vi "example_02_two_button.vi"() -> ()   [LabVIEW 2015, in "lv-dialog.lvlib" / "v1.lvlib"]
uses:
  v1.lvlib
  public/_controls/dialog_selection.ctl
  public/class/v1.lvclass
panel:
  in  "boolean_text_2":string="OK"
  in  "boolean_text_1":string="OK"
  in  "dialog_text":string="Press a button"
  out "error out":errorcluster
  out "dialog_selection":T1
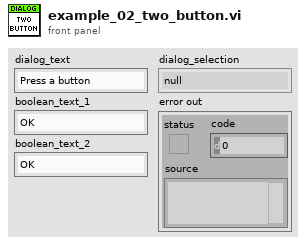
[diagram p1: front panel]
types:
  T1 = typedef "lv-dialog.lvlib/v1.lvlib/dialog_selection.ctl" = enum16{"null", "panel_closed", "button_1", "button_2", "button_3", "cancelled"}
  T2 = cluster{"dialog_text":string, "boolean_text_1":string, "boolean_text_2":string}
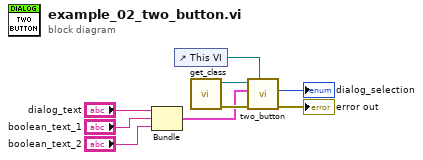
[diagram p0: block diagram]
diagram:
  n1 = Bundle("dialog_text"="dialog_text", "boolean_text_1"="boolean_text_1", "boolean_text_2"="boolean_text_2") -> (w3:T2)  [unwired: 1 in]
  n2 = control-ref of="This VI"() -> (w8:refnum<vi>)
  n3 = call "get_class.vi"() -> ("error out"=w9:errorcluster, "class"=w2:refnum<class "v1.lvclass">)  [unwired: 10 in]
  n4 = call-dynamic "two_button.vi"("callee"=w8, "error in (no error)"=w9, "configuration"=w3, "v1 in"=w2) -> ("error out"=→"error out":errorcluster, "dialog_selection"=→"dialog_selection":T1)  [unwired: 5 in, 1 out]
